vi "GenerateValveSequence.vi"(8 "Ctr Water Valve":u16(ring)=15 items=["A1", "A2", "A3", "A4", "B1", "B2", "B3", "B4", "B5", "B6", "B7", "B8", "A5", "A6", "A7", "A8"], 9 "Ctr Odor Valve":u16(ring)=14 items=["A1", "A2", "A3", "A4", "B1", "B2", "B3", "B4", "B5", "B6", "B7", "B8", "A5", "A6", "A7", "A8"], 11 "Mix Cluster":T3={"Ratio"=[0.6, 0.5], "Mix 2"=[12, 12], "Mix 1"=[0, 1]} {"Mix 1" items=["A1"=0, "A2"=1, "A3"=2, "A4"=3, "A5"=12]; "Mix 2" items=["B5"=8, "B6"=9, "B7"=10, "B8"=11, "A5"=12]}) -> (1 "Channel Sequence":T2(array[ring]), 2 "Flowboard Sequence":enum16{"A", "B", "C"}[][](array[ring]), 3 "Valve Sequence Data":T1(array[cluster]))   [LabVIEW 2016]
panel:
  in  "Flowboard":enum16{"A", "B", "C"}(ring)
  in  "Channel":enum16{"1", "2", "3", "4", "5", "6", "7", "8"}(ring)
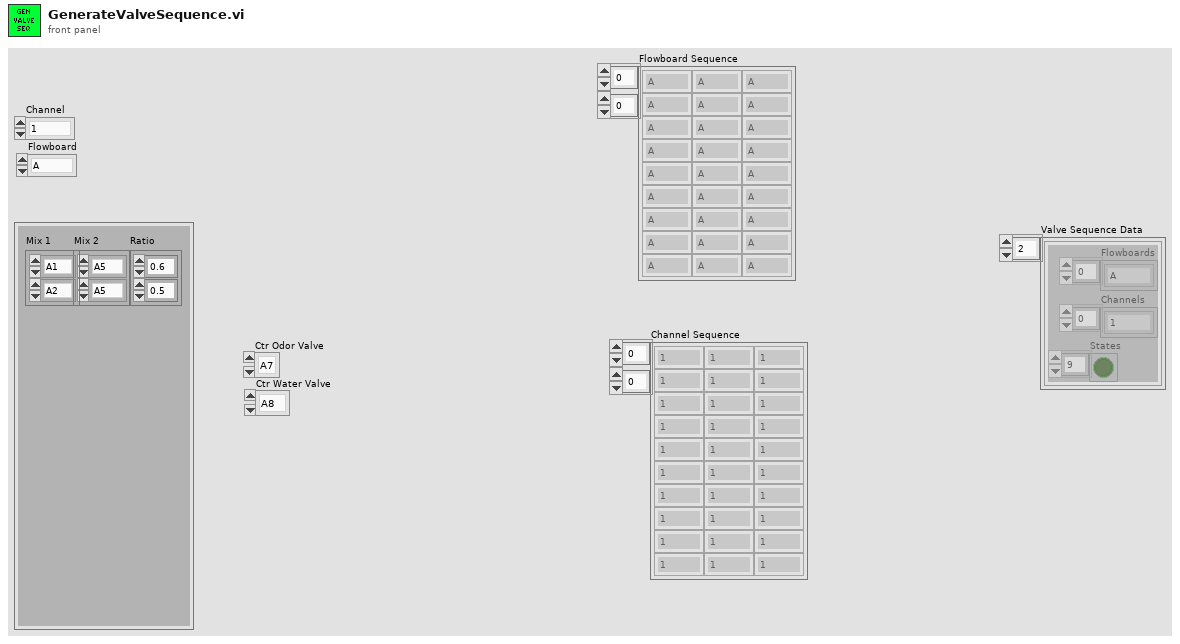
[diagram p1: front panel]
types:
  T1 = cluster{"Flowboards":enum16{"A", "B", "C"}[], "Channels":enum16{"1", "2", "3", "4", "5", "6", "7", "8"}[], "States":bool[]}[]
  T2 = enum16{"1", "2", "3", "4", "5", "6", "7", "8"}[][]
  T3 = cluster{"Ratio":dbl[], "Mix 2":u16[], "Mix 1":u16[]}
  T4 = cluster{"Flowboards":enum16{"A", "B", "C"}[], "Channels":enum16{"1", "2", "3", "4", "5", "6", "7", "8"}[], "States":bool[]}
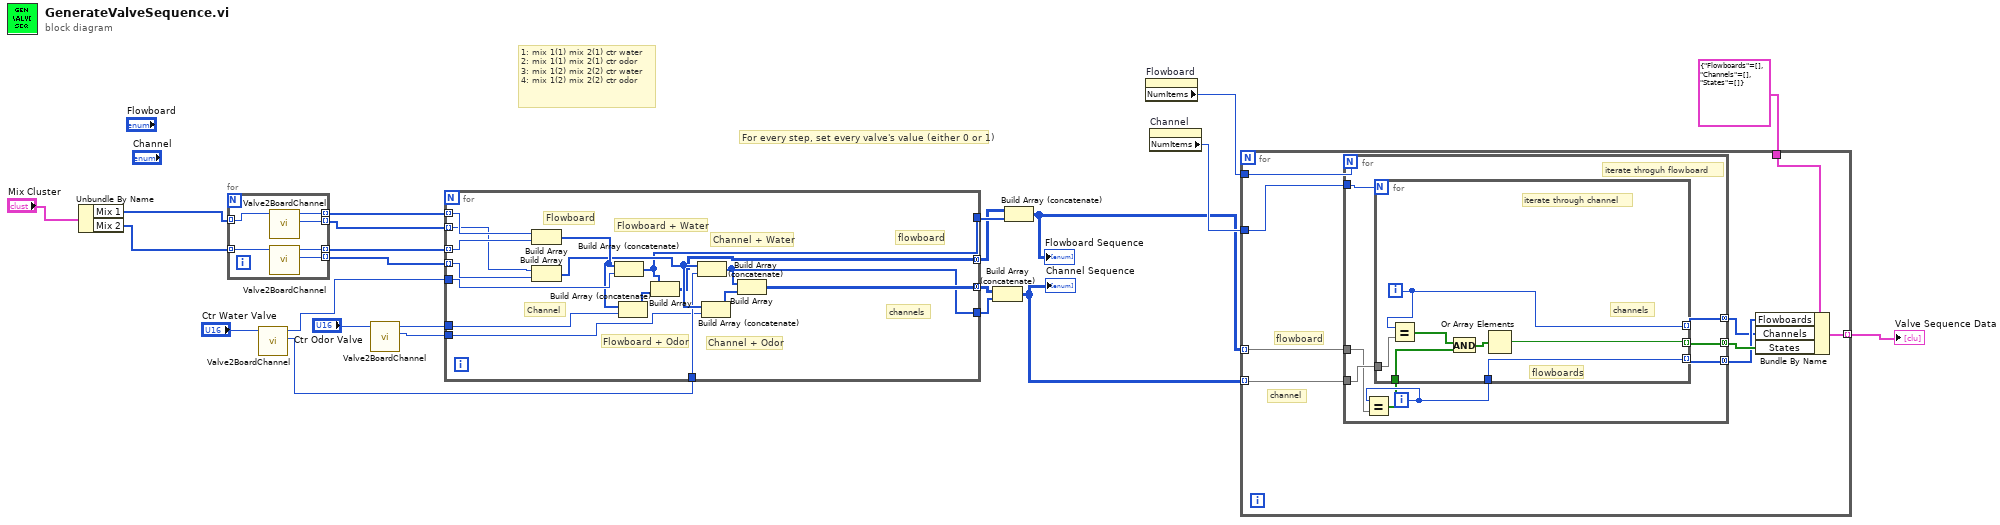
[diagram p0: block diagram]
diagram:
  # "1: mix 1(1) mix 2(1) ctr water\n2: mix 1(1) mix 2(1) ctr odor\n3: mix 1(2) mix 2(2) ctr water\n4: mix 1(2) mix 2(2) ctr odor"
  # "For every step, set every valve's value (either 0 or 1)"
  n1 = Unbundle By Name("Mix Cluster") -> ("Mix 1"=w20:u16[], "Mix 2"=w19:u16[])
  n2 = for {
    tunnel: w20 -> [w28] mode=indexing
    tunnel: w19 -> [w29] mode=indexing
    tunnel: [w27] -> w16 mode=indexing
    tunnel: [w26] -> w15 mode=indexing
    tunnel: [w25] -> w14 mode=indexing
    tunnel: [w24] -> w13 mode=indexing
    n3 = call "Valve2BoardChannel.vi"("ValveID"=w28) -> ("Channel"=w26:enum16{"1", "2", "3", "4", "5", "6", "7", "8"}, "Flowboard"=w27:enum16{"A", "B", "C"})  [unwired: 9 in]
    n4 = call "Valve2BoardChannel.vi"("ValveID"=w29) -> ("Channel"=w24:enum16{"1", "2", "3", "4", "5", "6", "7", "8"}, "Flowboard"=w25:enum16{"A", "B", "C"})  [unwired: 9 in]
  }
  n5 = call "Valve2BoardChannel.vi"("ValveID"="Ctr Water Valve") -> ("Channel"=w10:enum16{"1", "2", "3", "4", "5", "6", "7", "8"}, "Flowboard"=w12:enum16{"A", "B", "C"})  [unwired: 9 in]
  n6 = call "Valve2BoardChannel.vi"("ValveID"="Ctr Odor Valve") -> ("Channel"=w9:enum16{"1", "2", "3", "4", "5", "6", "7", "8"}, "Flowboard"=w11:enum16{"A", "B", "C"})  [unwired: 9 in]
  n7 = for {
    tunnel: w16 -> [w45] mode=indexing
    tunnel: w15 -> [w43] mode=indexing
    tunnel: w14 -> [w44] mode=indexing
    tunnel: w13 -> [w42] mode=indexing
    tunnel: w12 -> [w41]
    tunnel: w11 -> [w38]
    tunnel: w10 -> [w37]
    tunnel: w9 -> [w36]
    tunnel: [w33] -> w6 mode=concatenating
    tunnel: [w32] -> w7 mode=concatenating
    tunnel: [w31] -> w8
    tunnel: [w30] -> w5
    # "channels"
    # "flowboard"
    # "Channel + Odor"
    # "Channel + Water"
    # "Flowboard + Odor"
    # "Flowboard + Water"
    # "Channel"
    # "Flowboard"
    n8 = Build Array(w45, w44) -> (w40:enum16{"A", "B", "C"}[])
    n9 = Build Array(w43, w42) -> (w39:enum16{"1", "2", "3", "4", "5", "6", "7", "8"}[])
    n10 = Build Array (concatenate)(w40, w41) -> (w31:enum16{"A", "B", "C"}[])
    n11 = Build Array (concatenate)(w40, w38) -> (w35:enum16{"A", "B", "C"}[])
    n12 = Build Array(w31, w35) -> (w32:enum16{"A", "B", "C"}[][])
    n13 = Build Array (concatenate)(w39, w37) -> (w30:enum16{"1", "2", "3", "4", "5", "6", "7", "8"}[])
    n14 = Build Array (concatenate)(w39, w36) -> (w34:enum16{"1", "2", "3", "4", "5", "6", "7", "8"}[])
    n15 = Build Array(w30, w34) -> (w33:T2)
  }
  n16 = Build Array (concatenate)(w6, w5) -> (w3:T2)
  "Channel Sequence" <- w3
  n17 = Build Array (concatenate)(w7, w8) -> (w4:enum16{"A", "B", "C"}[][])
  "Flowboard Sequence" <- w4
  n18 = property on="Flowboard" class="Enum (strict)"() -> ("NumItems"=w18:u32)  [unwired: 2 in, 2 out]
  n19 = property on="Channel" class="Enum (strict)"() -> ("NumItems"=w17:u32)  [unwired: 2 in, 2 out]
  n20 = for {
    tunnel: w18 -> [w54]
    tunnel: w17 -> [w53]
    tunnel: w4 -> [w52] mode=indexing
    tunnel: w3 -> [w51] mode=indexing
    tunnel: T4 {"Flowboards"=[], "Channels"=[], "States"=[]} ("Valve Data") -> [w50]
    tunnel: [w46] -> w1 mode=indexing
    # "channel"
    # "flowboard"
    n21 = for {
      N: w54 -> [_]
      tunnel: w53 -> [w62]
      tunnel: [w61] -> w47 mode=concatenating
      tunnel: [w60] -> w48 mode=concatenating
      tunnel: w52 -> [w58]
      tunnel: w51 -> [w59]
      tunnel: [w55] -> w49 mode=concatenating
      i -> [w57]
      # "iterate throguh flowboard"
      n22 = Equal?(x=w57, y=w58) -> (x = y?=w56:bool[])
      n23 = for {
        N: w62 -> [_]
        tunnel: [w68] -> w61 mode=indexing
        tunnel: w57 -> [w67]
        tunnel: [w67] -> w60 mode=indexing
        tunnel: w59 -> [w69]
        tunnel: w56 -> [w65]
        tunnel: [w63] -> w55 mode=indexing
        i -> [w68]
        # "flowboards"
        # "channels"
        # "iterate through channel"
        n24 = Equal?(x=w68, y=w69) -> (x = y?=w66:bool[])
        n25 = And(x=w66, y=w65) -> (x .and. y?=w64:bool[])
        n26 = Or Array Elements(Boolean array=w64) -> (logical OR=w63:bool)
      }
    }
    n27 = Bundle By Name(cluster=w50, "Flowboards"=w48, "Channels"=w47, "States"=w49) -> (w46:T4)
  }
  "Valve Sequence Data" <- w1
